vi "String to Number.vi"(11 "whole match":string) -> (3 "Numeric":i32)   [LabVIEW 2022 SP3]
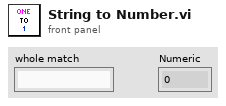
[diagram p1: front panel]
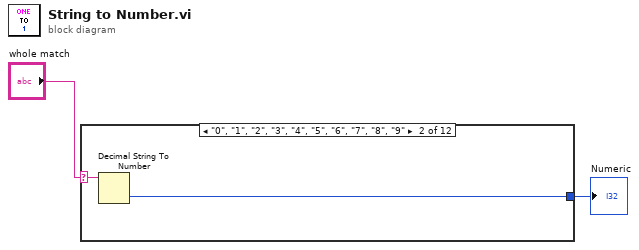
[diagram p0: block diagram]
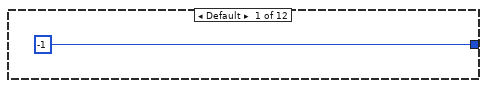
[diagram p2: hidden frame]
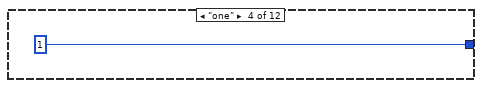
[diagram p4: hidden frame]
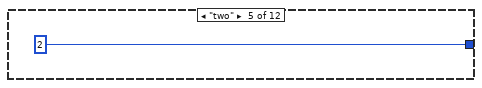
[diagram p5: hidden frame]
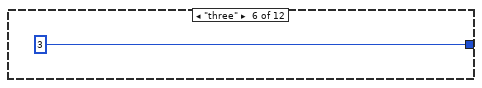
[diagram p6: hidden frame]
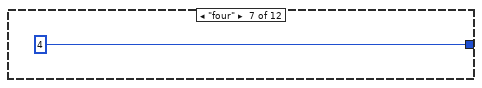
[diagram p7: hidden frame]
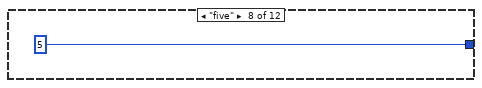
[diagram p8: hidden frame]
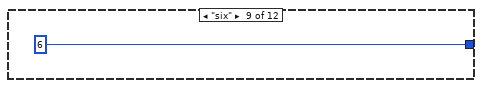
[diagram p9: hidden frame]
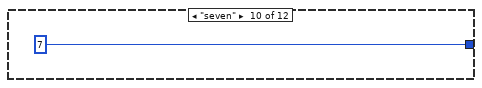
[diagram p10: hidden frame]
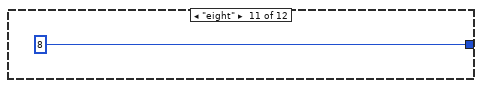
[diagram p11: hidden frame]
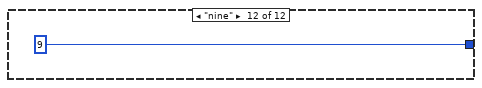
[diagram p12: hidden frame]
diagram:
  n1 = case shown="\"0\", \"1\", \"2\", \"3\", \"4\", \"5\", \"6\", \"7\", \"8\", \"9\"" "whole match" {
    selector: "whole match" -> [_ w5 _ _ _ _ _ _ _ _ _ _]
    tunnel: [-1 w4 _ 1 2 3 4 5 6 7 8 9] -> w2
    frame Default {
    }
    frame "0", "1", "2", "3", "4", "5", "6", "7", "8", "9" {
      n2 = Decimal String To Number(string=w5) -> (number=w4:i32)  [unwired: 2 in, 1 out]
    }
    frame "zero" {
    }
    frame "one" {
    }
    frame "two" {
    }
    frame "three" {
    }
    frame "four" {
    }
    frame "five" {
    }
    frame "six" {
    }
    frame "seven" {
    }
    frame "eight" {
    }
    frame "nine" {
    }
  }
  "Numeric" <- w2
